vi "十六进制显示转正常显示 (子VI).vi"(11 "字符串输入":string) -> (3 "字符串输出":string)   [LabVIEW 2016, in "环境动力监测库.lvlib"]
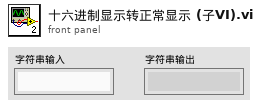
[diagram p1: front panel]
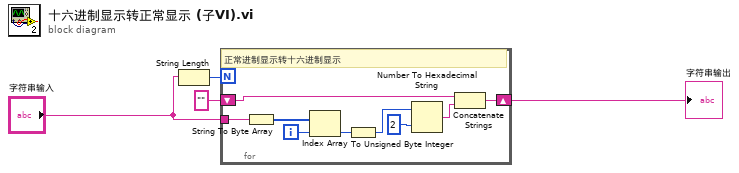
[diagram p0: block diagram]
diagram:
  n1 = String Length(string="字符串输入") -> (length=w4:i32)
  n2 = for {
    N: w4 -> [_]
    tunnel: "字符串输入" -> [w6]
    shift-right: [w13] -> w3
    shift-left: "" -> [w12]
    i -> [w5]
    # "正常进制显示转十六进制显示"
    n3 = String To Byte Array(string=w6) -> (unsigned byte array=w8:u8[])
    n4 = Index Array(array=w8, index=w5) -> (element=w9:u8)
    n5 = To Unsigned Byte Integer(number=w9) -> (unsigned 8bit integer=w10:u8)
    n6 = Number To Hexadecimal String(1:i16 2 ("宽度(-)"), 2:w10) -> (0:w7:string)
    n7 = Concatenate Strings(w12, w7) -> (w13:string)
  }
  "字符串输出" <- w3
